vi "Region-det-generate-Q-mat.vi"(8 "error in (no error)":errorcluster, 9 "Q region size JSON string":string="{\"regions\": [7, 8, 9, 10, 11, 12, 13, 14, 15, 16, 17, 18, 19, 20, 21, 22, 23, 24, 25, 26, 27, 28, 29, 30], \"7\": 1, \"8\": 2, \"9\": 2, \"10\": 2, \"11\": 2, \"12\": 2, \"13\": 2, \"14\": 2, \"15\": 2, \"16\": 2, \"17\": 3, \"18\": 4, \"19\": 6, \"20\": 8, \"21\": 9, \"22\": 11, \"23\": 12, \"24\": 13, \"25\": 15, \"26\": 16, \"27\": 17, \"28\": 18, \"29\": 20, \"30\": 20}", 10 "Q matrix JSON string":string="{\"7\": [[[12.153786444450104, -34.08974352571347], [-34.08974352571347, 87.34799155031487]]], \"8\": [[[4.10243439131574, -13.653163941582909], [-13.653163941582909, 35.53332337462381]], [[-12.153786444450104, 34.08974352571347], [34.08974352571347, -87.34799155031487]]], \"9\": [[[-4.10243439131574, 13.653163941582909], [13.653163941582909, -35.53332337462381]], [[2.229187499815464, -8.941787053410259], [-8.941787053410259, 23.76027041263613]]], \"10\": [[[-2.229187499815464, 8.941787053410259], [8.941787053410259, -23.76027041263613]], [[1.3522542136418623, -6.759181974052247], [-6.759181974052247, 18.42245047044422]]], \"11\": [[[-1.3522542136418623, 6.759181974052247], [6.759181974052247, -18.42245047044422]], [[0.8188029580326937, -5.441802783246412], [-5.441802783246412, 15.281707372952305]]], \"12\": [[[-0.8188029580326937, 5.441802783246412], [5.441802783246412, -15.281707372952305]], [[0.44486726637195817, -4.519994279916467], [-4.519994279916467, 13.139948191765672]]], \"13\": [[[-0.44486726637195817, 4.519994279916467], [4.519994279916467, -13.139948191765672]], [[0.15900921300751536, -3.8105885831447903], [-3.8105885831447903, 11.528446872578279]]], \"14\": [[[-0.15900921300751536, 3.8105885831447903], [3.8105885831447903, -11.528446872578279]], [[-0.07185075425810045, -3.228040009956443], [-3.228040009956443, 10.226903812813365]]], \"15\": [[[0.07185075425810045, 3.228040009956443], [3.228040009956443, -10.226903812813365]], [[-0.26471885527858824, -2.727690732778762], [-2.727690732778762, 9.118982088825604]]], \"16\": [[[0.26471885527858824, 2.727690732778762], [2.727690732778762, -9.118982088825604]], [[-0.42885400219319153, -2.2845911948651265], [-2.2845911948651265, 8.138393594102919]]], \"17\": [[[0.42885400219319153, 2.2845911948651265], [2.2845911948651265, -8.138393594102919]], [[-0.5693778392577464, -1.8843415109731665], [-1.8843415109731665, 7.2456112427105674]], [[0.26471885527858824, 2.727690732778762], [2.727690732778762, -9.118982088825604]]], \"18\": [[[0.42885400219319153, 2.2845911948651265], [2.2845911948651265, -8.138393594102919]], [[0.26471885527858824, 2.727690732778762], [2.727690732778762, -9.118982088825604]], [[0.5693778392577464, 1.8843415109731665], [1.8843415109731665, -7.2456112427105674]], [[-0.6890274698241711, -1.5186792347671538], [-1.5186792347671538, 6.416689238785417]]], \"19\": [[[0.07185075425810045, 3.228040009956443], [3.228040009956443, -10.226903812813365]], [[-0.7890948979502277, -1.1831617469595714], [-1.1831617469595714, 5.637448339860752]], [[0.6890274698241711, 1.5186792347671538], [1.5186792347671538, -6.416689238785417]], [[0.5693778392577464, 1.8843415109731665], [1.8843415109731665, -7.2456112427105674]], [[0.42885400219319153, 2.2845911948651265], [2.2845911948651265, -8.138393594102919]], [[0.26471885527858824, 2.727690732778762], [2.727690732778762, -9.118982088825604]]], \"20\": [[[0.07185075425810045, 3.228040009956443], [3.228040009956443, -10.226903812813365]], [[0.6890274698241711, 1.5186792347671538], [1.5186792347671538, -6.416689238785417]], [[0.26471885527858824, 2.727690732778762], [2.727690732778762, -9.118982088825604]], [[-0.15900921300751536, 3.8105885831447903], [3.8105885831447903, -11.528446872578279]], [[0.5693778392577464, 1.8843415109731665], [1.8843415109731665, -7.2456112427105674]], [[-0.8699869822867451, -0.8758477324242553], [-0.8758477324242553, 4.900249558737087]], [[0.42885400219319153, 2.2845911948651265], [2.2845911948651265, -8.138393594102919]], [[0.7890948979502277, 1.1831617469595714], [1.1831617469595714, -5.637448339860752]]], \"21\": [[[0.6890274698241711, 1.5186792347671538], [1.5186792347671538, -6.416689238785417]], [[0.5693778392577464, 1.8843415109731665], [1.8843415109731665, -7.2456112427105674]], [[0.07185075425810045, 3.228040009956443], [3.228040009956443, -10.226903812813365]], [[0.26471885527858824, 2.727690732778762], [2.727690732778762, -9.118982088825604]], [[-0.15900921300751536, 3.8105885831447903], [3.8105885831447903, -11.528446872578279]], [[0.42885400219319153, 2.2845911948651265], [2.2845911948651265, -8.138393594102919]], [[0.7890948979502277, 1.1831617469595714], [1.1831617469595714, -5.637448339860752]], [[0.8699869822867451, 0.8758477324242553], [0.8758477324242553, -4.900249558737087]], [[-0.9316079219101161, -0.5964745533197124], [-0.5964745533197124, 4.202092152988324]]], \"22\": [[[-0.44486726637195817, 4.519994279916467], [4.519994279916467, -13.139948191765672]], [[0.8699869822867451, 0.8758477324242553], [0.8758477324242553, -4.900249558737087]], [[0.7890948979502277, 1.1831617469595714], [1.1831617469595714, -5.637448339860752]], [[0.5693778392577464, 1.8843415109731665], [1.8843415109731665, -7.2456112427105674]], [[0.42885400219319153, 2.2845911948651265], [2.2845911948651265, -8.138393594102919]], [[0.26471885527858824, 2.727690732778762], [2.727690732778762, -9.118982088825604]], [[0.6890274698241711, 1.5186792347671538], [1.5186792347671538, -6.416689238785417]], [[0.9316079219101161, 0.5964745533197124], [0.5964745533197124, -4.202092152988324]], [[0.07185075425810045, 3.228040009956443], [3.228040009956443, -10.226903812813365]], [[-0.15900921300751536, 3.8105885831447903], [3.8105885831447903, -11.528446872578279]], [[-0.973669649597166, -0.3458747882987768], [-0.3458747882987768, 3.5434020949393448]]], \"23\": [[[0.6890274698241711, 1.5186792347671538], [1.5186792347671538, -6.416689238785417]], [[0.5693778392577464, 1.8843415109731665], [1.8843415109731665, -7.2456112427105674]], [[-0.15900921300751536, 3.8105885831447903], [3.8105885831447903, -11.528446872578279]], [[0.9316079219101161, 0.5964745533197124], [0.5964745533197124, -4.202092152988324]], [[-0.44486726637195817, 4.519994279916467], [4.519994279916467, -13.139948191765672]], [[-0.9959903650711946, -0.12548486438059792], [-0.12548486438059792, 2.927153336453356]], [[0.42885400219319153, 2.2845911948651265], [2.2845911948651265, -8.138393594102919]], [[0.07185075425810045, 3.228040009956443], [3.228040009956443, -10.226903812813365]], [[0.8699869822867451, 0.8758477324242553], [0.8758477324242553, -4.900249558737087]], [[0.26471885527858824, 2.727690732778762], [2.727690732778762, -9.118982088825604]], [[0.7890948979502277, 1.1831617469595714], [1.1831617469595714, -5.637448339860752]], [[0.973669649597166, 0.3458747882987768], [0.3458747882987768, -3.5434020949393448]]], \"24\": [[[-0.44486726637195817, 4.519994279916467], [4.519994279916467, -13.139948191765672]], [[0.8699869822867451, 0.8758477324242553], [0.8758477324242553, -4.900249558737087]], [[0.7890948979502277, 1.1831617469595714], [1.1831617469595714, -5.637448339860752]], [[0.973669649597166, 0.3458747882987768], [0.3458747882987768, -3.5434020949393448]], [[0.6890274698241711, 1.5186792347671538], [1.5186792347671538, -6.416689238785417]], [[-0.15900921300751536, 3.8105885831447903], [3.8105885831447903, -11.528446872578279]], [[0.9316079219101161, 0.5964745533197124], [0.5964745533197124, -4.202092152988324]], [[0.5693778392577464, 1.8843415109731665], [1.8843415109731665, -7.2456112427105674]], [[0.26471885527858824, 2.727690732778762], [2.727690732778762, -9.118982088825604]], [[0.42885400219319153, 2.2845911948651265], [2.2845911948651265, -8.138393594102919]], [[0.07185075425810045, 3.228040009956443], [3.228040009956443, -10.226903812813365]], [[0.9959903650711946, 0.12548486438059792], [0.12548486438059792, -2.927153336453356]], [[-0.9988125716968997, 0.06314653491524526], [0.06314653491524526, 2.3580847461628567]]], \"25\": [[[0.07185075425810045, 3.228040009956443], [3.228040009956443, -10.226903812813365]], [[0.9959903650711946, 0.12548486438059792], [0.12548486438059792, -2.927153336453356]], [[-0.15900921300751536, 3.8105885831447903], [3.8105885831447903, -11.528446872578279]], [[-0.44486726637195817, 4.519994279916467], [4.519994279916467, -13.139948191765672]], [[0.7890948979502277, 1.1831617469595714], [1.1831617469595714, -5.637448339860752]], [[0.973669649597166, 0.3458747882987768], [0.3458747882987768, -3.5434020949393448]], [[0.6890274698241711, 1.5186792347671538], [1.5186792347671538, -6.416689238785417]], [[-0.8188029580326937, 5.441802783246412], [5.441802783246412, -15.281707372952305]], [[0.5693778392577464, 1.8843415109731665], [1.8843415109731665, -7.2456112427105674]], [[0.8699869822867451, 0.8758477324242553], [0.8758477324242553, -4.900249558737087]], [[0.42885400219319153, 2.2845911948651265], [2.2845911948651265, -8.138393594102919]], [[0.9988125716968997, -0.06314653491524526], [-0.06314653491524526, -2.3580847461628567]], [[0.9316079219101161, 0.5964745533197124], [0.5964745533197124, -4.202092152988324]], [[-0.9831384435484145, 0.2189010734067785], [0.2189010734067785, 1.8418301760116593]], [[0.26471885527858824, 2.727690732778762], [2.727690732778762, -9.118982088825604]]], \"26\": [[[0.9988125716968997, -0.06314653491524526], [-0.06314653491524526, -2.3580847461628567]], [[0.7890948979502277, 1.1831617469595714], [1.1831617469595714, -5.637448339860752]], [[0.6890274698241711, 1.5186792347671538], [1.5186792347671538, -6.416689238785417]], [[-0.8188029580326937, 5.441802783246412], [5.441802783246412, -15.281707372952305]], [[0.973669649597166, 0.3458747882987768], [0.3458747882987768, -3.5434020949393448]], [[0.42885400219319153, 2.2845911948651265], [2.2845911948651265, -8.138393594102919]], [[0.9831384435484145, -0.2189010734067785], [-0.2189010734067785, -1.8418301760116593]], [[0.5693778392577464, 1.8843415109731665], [1.8843415109731665, -7.2456112427105674]], [[0.26471885527858824, 2.727690732778762], [2.727690732778762, -9.118982088825604]], [[-0.15900921300751536, 3.8105885831447903], [3.8105885831447903, -11.528446872578279]], [[0.07185075425810045, 3.228040009956443], [3.228040009956443, -10.226903812813365]], [[0.8699869822867451, 0.8758477324242553], [0.8758477324242553, -4.900249558737087]], [[-0.44486726637195817, 4.519994279916467], [4.519994279916467, -13.139948191765672]], [[-0.9510273469824555, 0.34167607911576714], [0.34167607911576714, 1.383831298624971]], [[0.9959903650711946, 0.12548486438059792], [0.12548486438059792, -2.927153336453356]], [[0.9316079219101161, 0.5964745533197124], [0.5964745533197124, -4.202092152988324]]], \"27\": [[[-0.15900921300751536, 3.8105885831447903], [3.8105885831447903, -11.528446872578279]], [[0.8699869822867451, 0.8758477324242553], [0.8758477324242553, -4.900249558737087]], [[0.9959903650711946, 0.12548486438059792], [0.12548486438059792, -2.927153336453356]], [[-0.44486726637195817, 4.519994279916467], [4.519994279916467, -13.139948191765672]], [[-0.8188029580326937, 5.441802783246412], [5.441802783246412, -15.281707372952305]], [[0.6890274698241711, 1.5186792347671538], [1.5186792347671538, -6.416689238785417]], [[0.973669649597166, 0.3458747882987768], [0.3458747882987768, -3.5434020949393448]], [[0.9988125716968997, -0.06314653491524526], [-0.06314653491524526, -2.3580847461628567]], [[0.5693778392577464, 1.8843415109731665], [1.8843415109731665, -7.2456112427105674]], [[0.9831384435484145, -0.2189010734067785], [-0.2189010734067785, -1.8418301760116593]], [[0.42885400219319153, 2.2845911948651265], [2.2845911948651265, -8.138393594102919]], [[0.26471885527858824, 2.727690732778762], [2.727690732778762, -9.118982088825604]], [[0.07185075425810045, 3.228040009956443], [3.228040009956443, -10.226903812813365]], [[0.9510273469824555, -0.34167607911576714], [-0.34167607911576714, -1.383831298624971]], [[0.9316079219101161, 0.5964745533197124], [0.5964745533197124, -4.202092152988324]], [[-0.9057306306783274, 0.43290837829811324], [0.43290837829811324, 0.9880228896112502]], [[0.7890948979502277, 1.1831617469595714], [1.1831617469595714, -5.637448339860752]]], \"28\": [[[0.9988125716968997, -0.06314653491524526], [-0.06314653491524526, -2.3580847461628567]], [[0.7890948979502277, 1.1831617469595714], [1.1831617469595714, -5.637448339860752]], [[0.6890274698241711, 1.5186792347671538], [1.5186792347671538, -6.416689238785417]], [[0.9057306306783274, -0.43290837829811324], [-0.43290837829811324, -0.9880228896112502]], [[0.9959903650711946, 0.12548486438059792], [0.12548486438059792, -2.927153336453356]], [[0.42885400219319153, 2.2845911948651265], [2.2845911948651265, -8.138393594102919]], [[-1.0590591425483402, 0.6166854883494433], [0.6166854883494433, 0.8153035123264498]], [[0.5693778392577464, 1.8843415109731665], [1.8843415109731665, -7.2456112427105674]], [[0.8699869822867451, 0.8758477324242553], [0.8758477324242553, -4.900249558737087]], [[0.26471885527858824, 2.727690732778762], [2.727690732778762, -9.118982088825604]], [[-0.15900921300751536, 3.8105885831447903], [3.8105885831447903, -11.528446872578279]], [[-0.44486726637195817, 4.519994279916467], [4.519994279916467, -13.139948191765672]], [[0.07185075425810045, 3.228040009956443], [3.228040009956443, -10.226903812813365]], [[-0.8188029580326937, 5.441802783246412], [5.441802783246412, -15.281707372952305]], [[0.9831384435484145, -0.2189010734067785], [-0.2189010734067785, -1.8418301760116593]], [[0.973669649597166, 0.3458747882987768], [0.3458747882987768, -3.5434020949393448]], [[0.9510273469824555, -0.34167607911576714], [-0.34167607911576714, -1.383831298624971]], [[0.9316079219101161, 0.5964745533197124], [0.5964745533197124, -4.202092152988324]]], \"29\": [[[-0.15900921300751536, 3.8105885831447903], [3.8105885831447903, -11.528446872578279]], [[0.9831384435484145, -0.2189010734067785], [-0.2189010734067785, -1.8418301760116593]], [[0.9510273469824555, -0.34167607911576714], [-0.34167607911576714, -1.383831298624971]], [[0.9057306306783274, -0.43290837829811324], [-0.43290837829811324, -0.9880228896112502]], [[-0.8188029580326937, 5.441802783246412], [5.441802783246412, -15.281707372952305]], [[-1.3522542136418623, 6.759181974052247], [6.759181974052247, -18.42245047044422]], [[0.6890274698241711, 1.5186792347671538], [1.5186792347671538, -6.416689238785417]], [[-0.44486726637195817, 4.519994279916467], [4.519994279916467, -13.139948191765672]], [[0.9988125716968997, -0.06314653491524526], [-0.06314653491524526, -2.3580847461628567]], [[0.42885400219319153, 2.2845911948651265], [2.2845911948651265, -8.138393594102919]], [[0.26471885527858824, 2.727690732778762], [2.727690732778762, -9.118982088825604]], [[0.973669649597166, 0.3458747882987768], [0.3458747882987768, -3.5434020949393448]], [[0.07185075425810045, 3.228040009956443], [3.228040009956443, -10.226903812813365]], [[0.8699869822867451, 0.8758477324242553], [0.8758477324242553, -4.900249558737087]], [[0.7890948979502277, 1.1831617469595714], [1.1831617469595714, -5.637448339860752]], [[0.5693778392577464, 1.8843415109731665], [1.8843415109731665, -7.2456112427105674]], [[1.0590591425483402, -0.6166854883494433], [-0.6166854883494433, -0.8153035123264498]], [[0.9316079219101161, 0.5964745533197124], [0.5964745533197124, -4.202092152988324]], [[-1.3422949248000238, 0.9059207832310605], [0.9059207832310605, 0.6496203544649515]], [[0.9959903650711946, 0.12548486438059792], [0.12548486438059792, -2.927153336453356]]], \"30\": [[[0.07185075425810045, 3.228040009956443], [3.228040009956443, -10.226903812813365]], [[-0.15900921300751536, 3.8105885831447903], [3.8105885831447903, -11.528446872578279]], [[-0.8188029580326937, 5.441802783246412], [5.441802783246412, -15.281707372952305]], [[0.9057306306783274, -0.43290837829811324], [-0.43290837829811324, -0.9880228896112502]], [[0.6890274698241711, 1.5186792347671538], [1.5186792347671538, -6.416689238785417]], [[1.0590591425483402, -0.6166854883494433], [-0.6166854883494433, -0.8153035123264498]], [[0.9510273469824555, -0.34167607911576714], [-0.34167607911576714, -1.383831298624971]], [[0.5693778392577464, 1.8843415109731665], [1.8843415109731665, -7.2456112427105674]], [[0.9959903650711946, 0.12548486438059792], [0.12548486438059792, -2.927153336453356]], [[0.26471885527858824, 2.727690732778762], [2.727690732778762, -9.118982088825604]], [[-0.44486726637195817, 4.519994279916467], [4.519994279916467, -13.139948191765672]], [[0.9831384435484145, -0.2189010734067785], [-0.2189010734067785, -1.8418301760116593]], [[0.7890948979502277, 1.1831617469595714], [1.1831617469595714, -5.637448339860752]], [[1.3422949248000238, -0.9059207832310605], [-0.9059207832310605, -0.6496203544649515]], [[0.42885400219319153, 2.2845911948651265], [2.2845911948651265, -8.138393594102919]], [[-1.3522542136418623, 6.759181974052247], [6.759181974052247, -18.42245047044422]], [[0.9316079219101161, 0.5964745533197124], [0.5964745533197124, -4.202092152988324]], [[0.9988125716968997, -0.06314653491524526], [-0.06314653491524526, -2.3580847461628567]], [[0.973669649597166, 0.3458747882987768], [0.3458747882987768, -3.5434020949393448]], [[0.8699869822867451, 0.8758477324242553], [0.8758477324242553, -4.900249558737087]]]}") -> (0 "error out":errorcluster, 1 "Q Matrices":dbl[][][][](array[numeric]), 2 "Index array":dbl[](array[numeric]), 3 "Regions":i32[](array[numeric]))   [LabVIEW 2016]
panel:
  # "This objective of this piece of code is the following:\n- A bunch of arrays of Q matrices is generated corresponding to each region of the state space\n- An \"index array\" is generated which stores the index of the region in the Q matrix array at the index of the \"index array\"\n(i.e. if the region array has \"7\", \"8\", \"9\", the index array will have elements 0 at index 7, 1 at 8, and 2 at 9 - this is because \nLabVIEW does not support maps)"
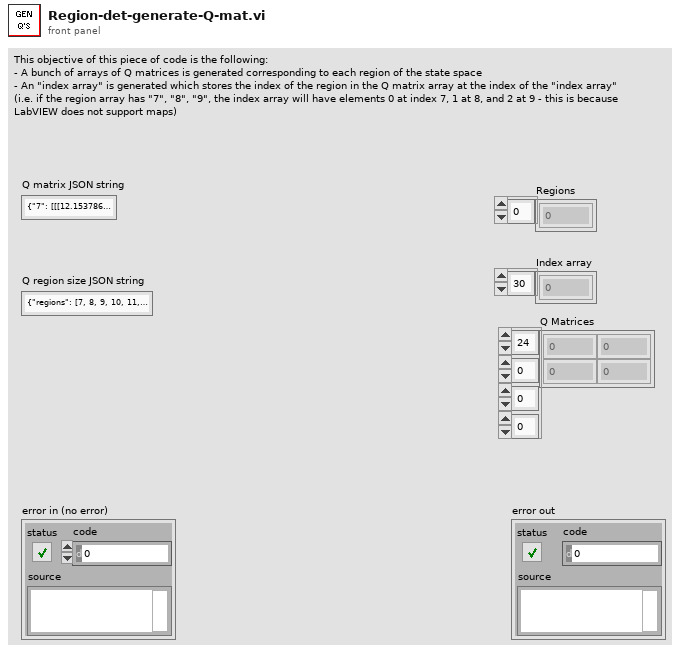
[diagram p1: front panel]
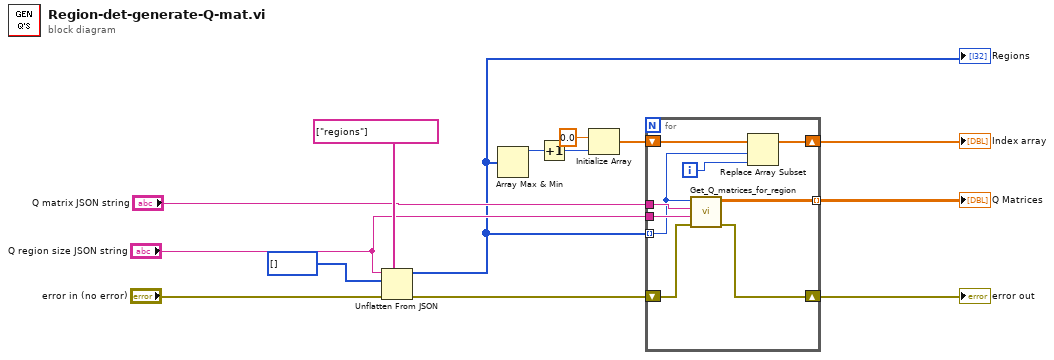
[diagram p0: block diagram]
diagram:
  n1 = Unflatten From JSON(path=string[] ["regions"], JSON string="Q region size JSON string", type and defaults=i32[] [], error in (no error)="error in (no error)") -> (value=w8:i32[], error out=w2:errorcluster)  [unwired: 3 in]
  "Regions" <- w8
  n2 = Array Max & Min(array=w8) -> (max value=w6:i32)  [unwired: 3 out]
  n3 = Increment(x=w6) -> (x+1=w5:i32)
  n4 = Initialize Array(0.0 ("element"), w5) -> (w7:dbl[])
  n5 = for {
    tunnel: w8 -> [w19] mode=indexing
    tunnel: "Q matrix JSON string" -> [w23]
    tunnel: "Q region size JSON string" -> [w22]
    tunnel: [w21] -> w10 mode=indexing
    shift-right: [w18] -> w4
    shift-left: w7 -> [w20]
    shift-right: [w16] -> w1
    shift-left: w2 -> [w17]
    i -> [w15]
    n6 = call "Get_Q_matrices_for_region.vi"("error in (no error)"=w17, "Q region size JSON string"=w22, "Q matrix JSON string"=w23, "Region"=w19) -> ("error out"=w16:errorcluster, "Q Matrices"=w21:dbl[][][])  [unwired: 6 in]
    n7 = Replace Array Subset(array=w20, new element=w15, index=w19) -> (w18:dbl[])
  }
  "Q Matrices" <- w10
  "Index array" <- w4
  "error out" <- w1
